vi "Normal.vi"() -> (0 "高難度挑戰":bool)   [LabVIEW 2014]
uses:
  <vilib>/Utility/inputDevices.llb/keyboardAcquire.vi
  <vilib>/Utility/inputDevices.llb/closeKeyboard.vi
panel:
  out "Å]YÄ²":i32
  out "Å]XÄ²":i32
  out "Å]Vy":i64
  out "Å]Vx":i32
  out "魔王":bool
  out "終點":bool
  out "遊玩時間":i32
  out "X障礙":bool
  out "Y位置 2":i32
  out "x位置 2":i32
  out "X":dbl
  out "Y":dbl
  out "小精靈":bool
  out "x位置":i32
  out "Y位置":i32
  out "Y障礙":bool
  out "x觸及位置":i32
  out "y觸及位置":i32
  out "x-y":u32
  out "Vy":i32
  out "Vx":i32
  # "小精靈"
  # "500"
  # "障礙"
  # "400"
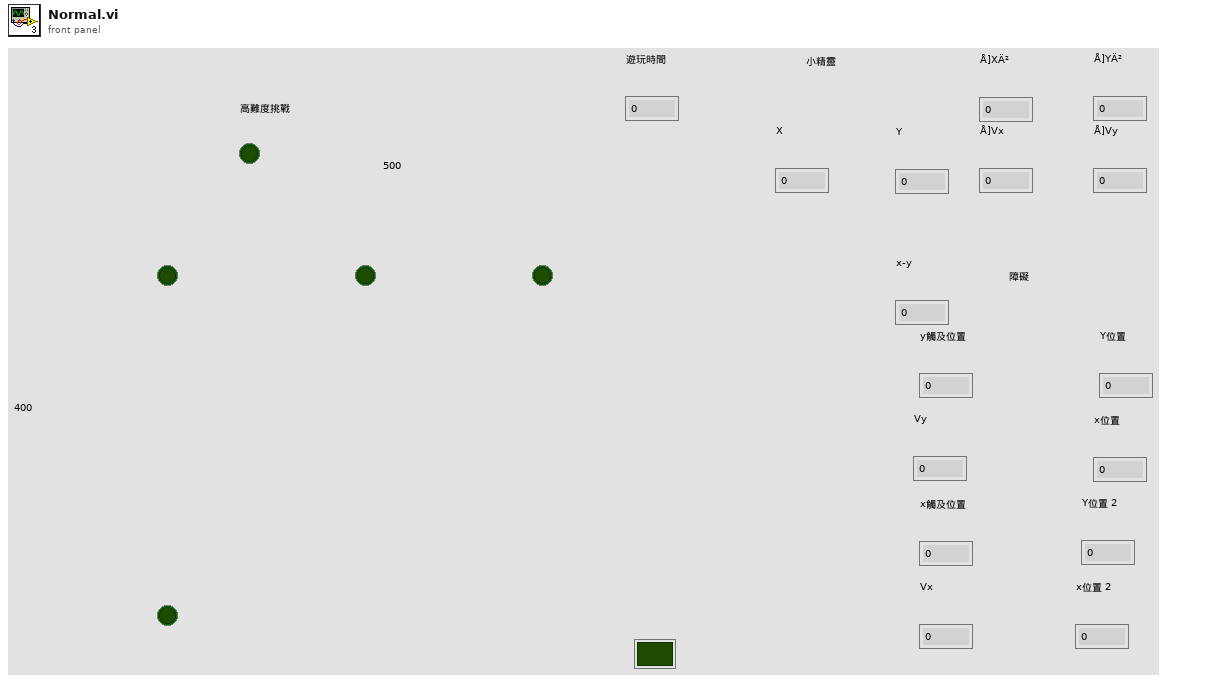
[diagram p1: front panel]
types:
  T1 = enum16{"0", "1", "2", "3", "4", "5", "6", "7", "8", "9", "A", "B", "C", "D", "E", "F", "G", "H", "I", "J", "K", "L", "M", "N", "O", "P", "Q", "R", "S", "T", "U", "V", "W", "X", "Y", "Z", "F1", "F2", "F3", "F4", "F5", "F6", "F7", "F8", "F9", "F10", "F11", "F12", "F13", "F14", "F15", "ADD", "BACK", "BACKSLASH", "CAPITAL", "COMMA", "DECIMAL", "DELETE", "DIVIDE", "DOWN", "END", "EQUALS", "ESCAPE", "GRAVE (`)", "HOME", "INSERT", "LBRACKET", "LCONTROL", "LEFT", "L ALT", "LSHIFT", "LWIN", "MINUS", "MULTIPLY", "NEXT", "NUMLOCK", "NUMPAD_0", "NUMPAD_1", "NUMPAD_2", "NUMPAD_3", "NUMPAD_4", "NUMPAD_5", "NUMPAD_6", "NUMPAD_7", "NUMPAD_8", "NUMPAD_9", "PAUSE", "PERIOD", "PRIOR (PG UP)", "RBRACKET", "RCONTROL", "RETURN", "RIGHT", "R ALT", "RSHIFT", "RWIN", "SCROLL", "SEMICOLON", "SLASH", "SPACE", "SUBTRACT", "TAB", "UP", "ENTER (num pad)", "' (quote)"}[]
  T2 = cluster{"keys pressed[0]":enum16{"0", "1", "2", "3", "4", "5", "6", "7", "8", "9", "A", "B", "C", "D", "E", "F", "G", "H", "I", "J", "K", "L", "M", "N", "O", "P", "Q", "R", "S", "T", "U", "V", "W", "X", "Y", "Z", "F1", "F2", "F3", "F4", "F5", "F6", "F7", "F8", "F9", "F10", "F11", "F12", "F13", "F14", "F15", "ADD", "BACK", "BACKSLASH", "CAPITAL", "COMMA", "DECIMAL", "DELETE", "DIVIDE", "DOWN", "END", "EQUALS", "ESCAPE", "GRAVE (`)", "HOME", "INSERT", "LBRACKET", "LCONTROL", "LEFT", "L ALT", "LSHIFT", "LWIN", "MINUS", "MULTIPLY", "NEXT", "NUMLOCK", "NUMPAD_0", "NUMPAD_1", "NUMPAD_2", "NUMPAD_3", "NUMPAD_4", "NUMPAD_5", "NUMPAD_6", "NUMPAD_7", "NUMPAD_8", "NUMPAD_9", "PAUSE", "PERIOD", "PRIOR (PG UP)", "RBRACKET", "RCONTROL", "RETURN", "RIGHT", "R ALT", "RSHIFT", "RWIN", "SCROLL", "SEMICOLON", "SLASH", "SPACE", "SUBTRACT", "TAB", "UP", "ENTER (num pad)", "' (quote)"}, "keys pressed[1]":enum16{"0", "1", "2", "3", "4", "5", "6", "7", "8", "9", "A", "B", "C", "D", "E", "F", "G", "H", "I", "J", "K", "L", "M", "N", "O", "P", "Q", "R", "S", "T", "U", "V", "W", "X", "Y", "Z", "F1", "F2", "F3", "F4", "F5", "F6", "F7", "F8", "F9", "F10", "F11", "F12", "F13", "F14", "F15", "ADD", "BACK", "BACKSLASH", "CAPITAL", "COMMA", "DECIMAL", "DELETE", "DIVIDE", "DOWN", "END", "EQUALS", "ESCAPE", "GRAVE (`)", "HOME", "INSERT", "LBRACKET", "LCONTROL", "LEFT", "L ALT", "LSHIFT", "LWIN", "MINUS", "MULTIPLY", "NEXT", "NUMLOCK", "NUMPAD_0", "NUMPAD_1", "NUMPAD_2", "NUMPAD_3", "NUMPAD_4", "NUMPAD_5", "NUMPAD_6", "NUMPAD_7", "NUMPAD_8", "NUMPAD_9", "PAUSE", "PERIOD", "PRIOR (PG UP)", "RBRACKET", "RCONTROL", "RETURN", "RIGHT", "R ALT", "RSHIFT", "RWIN", "SCROLL", "SEMICOLON", "SLASH", "SPACE", "SUBTRACT", "TAB", "UP", "ENTER (num pad)", "' (quote)"}, "keys pressed[2]":enum16{"0", "1", "2", "3", "4", "5", "6", "7", "8", "9", "A", "B", "C", "D", "E", "F", "G", "H", "I", "J", "K", "L", "M", "N", "O", "P", "Q", "R", "S", "T", "U", "V", "W", "X", "Y", "Z", "F1", "F2", "F3", "F4", "F5", "F6", "F7", "F8", "F9", "F10", "F11", "F12", "F13", "F14", "F15", "ADD", "BACK", "BACKSLASH", "CAPITAL", "COMMA", "DECIMAL", "DELETE", "DIVIDE", "DOWN", "END", "EQUALS", "ESCAPE", "GRAVE (`)", "HOME", "INSERT", "LBRACKET", "LCONTROL", "LEFT", "L ALT", "LSHIFT", "LWIN", "MINUS", "MULTIPLY", "NEXT", "NUMLOCK", "NUMPAD_0", "NUMPAD_1", "NUMPAD_2", "NUMPAD_3", "NUMPAD_4", "NUMPAD_5", "NUMPAD_6", "NUMPAD_7", "NUMPAD_8", "NUMPAD_9", "PAUSE", "PERIOD", "PRIOR (PG UP)", "RBRACKET", "RCONTROL", "RETURN", "RIGHT", "R ALT", "RSHIFT", "RWIN", "SCROLL", "SEMICOLON", "SLASH", "SPACE", "SUBTRACT", "TAB", "UP", "ENTER (num pad)", "' (quote)"}, "keys pressed[3]":enum16{"0", "1", "2", "3", "4", "5", "6", "7", "8", "9", "A", "B", "C", "D", "E", "F", "G", "H", "I", "J", "K", "L", "M", "N", "O", "P", "Q", "R", "S", "T", "U", "V", "W", "X", "Y", "Z", "F1", "F2", "F3", "F4", "F5", "F6", "F7", "F8", "F9", "F10", "F11", "F12", "F13", "F14", "F15", "ADD", "BACK", "BACKSLASH", "CAPITAL", "COMMA", "DECIMAL", "DELETE", "DIVIDE", "DOWN", "END", "EQUALS", "ESCAPE", "GRAVE (`)", "HOME", "INSERT", "LBRACKET", "LCONTROL", "LEFT", "L ALT", "LSHIFT", "LWIN", "MINUS", "MULTIPLY", "NEXT", "NUMLOCK", "NUMPAD_0", "NUMPAD_1", "NUMPAD_2", "NUMPAD_3", "NUMPAD_4", "NUMPAD_5", "NUMPAD_6", "NUMPAD_7", "NUMPAD_8", "NUMPAD_9", "PAUSE", "PERIOD", "PRIOR (PG UP)", "RBRACKET", "RCONTROL", "RETURN", "RIGHT", "R ALT", "RSHIFT", "RWIN", "SCROLL", "SEMICOLON", "SLASH", "SPACE", "SUBTRACT", "TAB", "UP", "ENTER (num pad)", "' (quote)"}, "keys pressed[4]":enum16{"0", "1", "2", "3", "4", "5", "6", "7", "8", "9", "A", "B", "C", "D", "E", "F", "G", "H", "I", "J", "K", "L", "M", "N", "O", "P", "Q", "R", "S", "T", "U", "V", "W", "X", "Y", "Z", "F1", "F2", "F3", "F4", "F5", "F6", "F7", "F8", "F9", "F10", "F11", "F12", "F13", "F14", "F15", "ADD", "BACK", "BACKSLASH", "CAPITAL", "COMMA", "DECIMAL", "DELETE", "DIVIDE", "DOWN", "END", "EQUALS", "ESCAPE", "GRAVE (`)", "HOME", "INSERT", "LBRACKET", "LCONTROL", "LEFT", "L ALT", "LSHIFT", "LWIN", "MINUS", "MULTIPLY", "NEXT", "NUMLOCK", "NUMPAD_0", "NUMPAD_1", "NUMPAD_2", "NUMPAD_3", "NUMPAD_4", "NUMPAD_5", "NUMPAD_6", "NUMPAD_7", "NUMPAD_8", "NUMPAD_9", "PAUSE", "PERIOD", "PRIOR (PG UP)", "RBRACKET", "RCONTROL", "RETURN", "RIGHT", "R ALT", "RSHIFT", "RWIN", "SCROLL", "SEMICOLON", "SLASH", "SPACE", "SUBTRACT", "TAB", "UP", "ENTER (num pad)", "' (quote)"}, "keys pressed[5]":enum16{"0", "1", "2", "3", "4", "5", "6", "7", "8", "9", "A", "B", "C", "D", "E", "F", "G", "H", "I", "J", "K", "L", "M", "N", "O", "P", "Q", "R", "S", "T", "U", "V", "W", "X", "Y", "Z", "F1", "F2", "F3", "F4", "F5", "F6", "F7", "F8", "F9", "F10", "F11", "F12", "F13", "F14", "F15", "ADD", "BACK", "BACKSLASH", "CAPITAL", "COMMA", "DECIMAL", "DELETE", "DIVIDE", "DOWN", "END", "EQUALS", "ESCAPE", "GRAVE (`)", "HOME", "INSERT", "LBRACKET", "LCONTROL", "LEFT", "L ALT", "LSHIFT", "LWIN", "MINUS", "MULTIPLY", "NEXT", "NUMLOCK", "NUMPAD_0", "NUMPAD_1", "NUMPAD_2", "NUMPAD_3", "NUMPAD_4", "NUMPAD_5", "NUMPAD_6", "NUMPAD_7", "NUMPAD_8", "NUMPAD_9", "PAUSE", "PERIOD", "PRIOR (PG UP)", "RBRACKET", "RCONTROL", "RETURN", "RIGHT", "R ALT", "RSHIFT", "RWIN", "SCROLL", "SEMICOLON", "SLASH", "SPACE", "SUBTRACT", "TAB", "UP", "ENTER (num pad)", "' (quote)"}, "keys pressed[6]":enum16{"0", "1", "2", "3", "4", "5", "6", "7", "8", "9", "A", "B", "C", "D", "E", "F", "G", "H", "I", "J", "K", "L", "M", "N", "O", "P", "Q", "R", "S", "T", "U", "V", "W", "X", "Y", "Z", "F1", "F2", "F3", "F4", "F5", "F6", "F7", "F8", "F9", "F10", "F11", "F12", "F13", "F14", "F15", "ADD", "BACK", "BACKSLASH", "CAPITAL", "COMMA", "DECIMAL", "DELETE", "DIVIDE", "DOWN", "END", "EQUALS", "ESCAPE", "GRAVE (`)", "HOME", "INSERT", "LBRACKET", "LCONTROL", "LEFT", "L ALT", "LSHIFT", "LWIN", "MINUS", "MULTIPLY", "NEXT", "NUMLOCK", "NUMPAD_0", "NUMPAD_1", "NUMPAD_2", "NUMPAD_3", "NUMPAD_4", "NUMPAD_5", "NUMPAD_6", "NUMPAD_7", "NUMPAD_8", "NUMPAD_9", "PAUSE", "PERIOD", "PRIOR (PG UP)", "RBRACKET", "RCONTROL", "RETURN", "RIGHT", "R ALT", "RSHIFT", "RWIN", "SCROLL", "SEMICOLON", "SLASH", "SPACE", "SUBTRACT", "TAB", "UP", "ENTER (num pad)", "' (quote)"}, "keys pressed[7]":enum16{"0", "1", "2", "3", "4", "5", "6", "7", "8", "9", "A", "B", "C", "D", "E", "F", "G", "H", "I", "J", "K", "L", "M", "N", "O", "P", "Q", "R", "S", "T", "U", "V", "W", "X", "Y", "Z", "F1", "F2", "F3", "F4", "F5", "F6", "F7", "F8", "F9", "F10", "F11", "F12", "F13", "F14", "F15", "ADD", "BACK", "BACKSLASH", "CAPITAL", "COMMA", "DECIMAL", "DELETE", "DIVIDE", "DOWN", "END", "EQUALS", "ESCAPE", "GRAVE (`)", "HOME", "INSERT", "LBRACKET", "LCONTROL", "LEFT", "L ALT", "LSHIFT", "LWIN", "MINUS", "MULTIPLY", "NEXT", "NUMLOCK", "NUMPAD_0", "NUMPAD_1", "NUMPAD_2", "NUMPAD_3", "NUMPAD_4", "NUMPAD_5", "NUMPAD_6", "NUMPAD_7", "NUMPAD_8", "NUMPAD_9", "PAUSE", "PERIOD", "PRIOR (PG UP)", "RBRACKET", "RCONTROL", "RETURN", "RIGHT", "R ALT", "RSHIFT", "RWIN", "SCROLL", "SEMICOLON", "SLASH", "SPACE", "SUBTRACT", "TAB", "UP", "ENTER (num pad)", "' (quote)"}, "keys pressed[8]":enum16{"0", "1", "2", "3", "4", "5", "6", "7", "8", "9", "A", "B", "C", "D", "E", "F", "G", "H", "I", "J", "K", "L", "M", "N", "O", "P", "Q", "R", "S", "T", "U", "V", "W", "X", "Y", "Z", "F1", "F2", "F3", "F4", "F5", "F6", "F7", "F8", "F9", "F10", "F11", "F12", "F13", "F14", "F15", "ADD", "BACK", "BACKSLASH", "CAPITAL", "COMMA", "DECIMAL", "DELETE", "DIVIDE", "DOWN", "END", "EQUALS", "ESCAPE", "GRAVE (`)", "HOME", "INSERT", "LBRACKET", "LCONTROL", "LEFT", "L ALT", "LSHIFT", "LWIN", "MINUS", "MULTIPLY", "NEXT", "NUMLOCK", "NUMPAD_0", "NUMPAD_1", "NUMPAD_2", "NUMPAD_3", "NUMPAD_4", "NUMPAD_5", "NUMPAD_6", "NUMPAD_7", "NUMPAD_8", "NUMPAD_9", "PAUSE", "PERIOD", "PRIOR (PG UP)", "RBRACKET", "RCONTROL", "RETURN", "RIGHT", "R ALT", "RSHIFT", "RWIN", "SCROLL", "SEMICOLON", "SLASH", "SPACE", "SUBTRACT", "TAB", "UP", "ENTER (num pad)", "' (quote)"}}
  T3 = enum16{"0", "1", "2", "3", "4", "5", "6", "7", "8", "9", "A", "B", "C", "D", "E", "F", "G", "H", "I", "J", "K", "L", "M", "N", "O", "P", "Q", "R", "S", "T", "U", "V", "W", "X", "Y", "Z", "F1", "F2", "F3", "F4", "F5", "F6", "F7", "F8", "F9", "F10", "F11", "F12", "F13", "F14", "F15", "ADD", "BACK", "BACKSLASH", "CAPITAL", "COMMA", "DECIMAL", "DELETE", "DIVIDE", "DOWN", "END", "EQUALS", "ESCAPE", "GRAVE (`)", "HOME", "INSERT", "LBRACKET", "LCONTROL", "LEFT", "L ALT", "LSHIFT", "LWIN", "MINUS", "MULTIPLY", "NEXT", "NUMLOCK", "NUMPAD_0", "NUMPAD_1", "NUMPAD_2", "NUMPAD_3", "NUMPAD_4", "NUMPAD_5", "NUMPAD_6", "NUMPAD_7", "NUMPAD_8", "NUMPAD_9", "PAUSE", "PERIOD", "PRIOR (PG UP)", "RBRACKET", "RCONTROL", "RETURN", "RIGHT", "R ALT", "RSHIFT", "RWIN", "SCROLL", "SEMICOLON", "SLASH", "SPACE", "SUBTRACT", "TAB", "UP", "ENTER (num pad)", "' (quote)"}
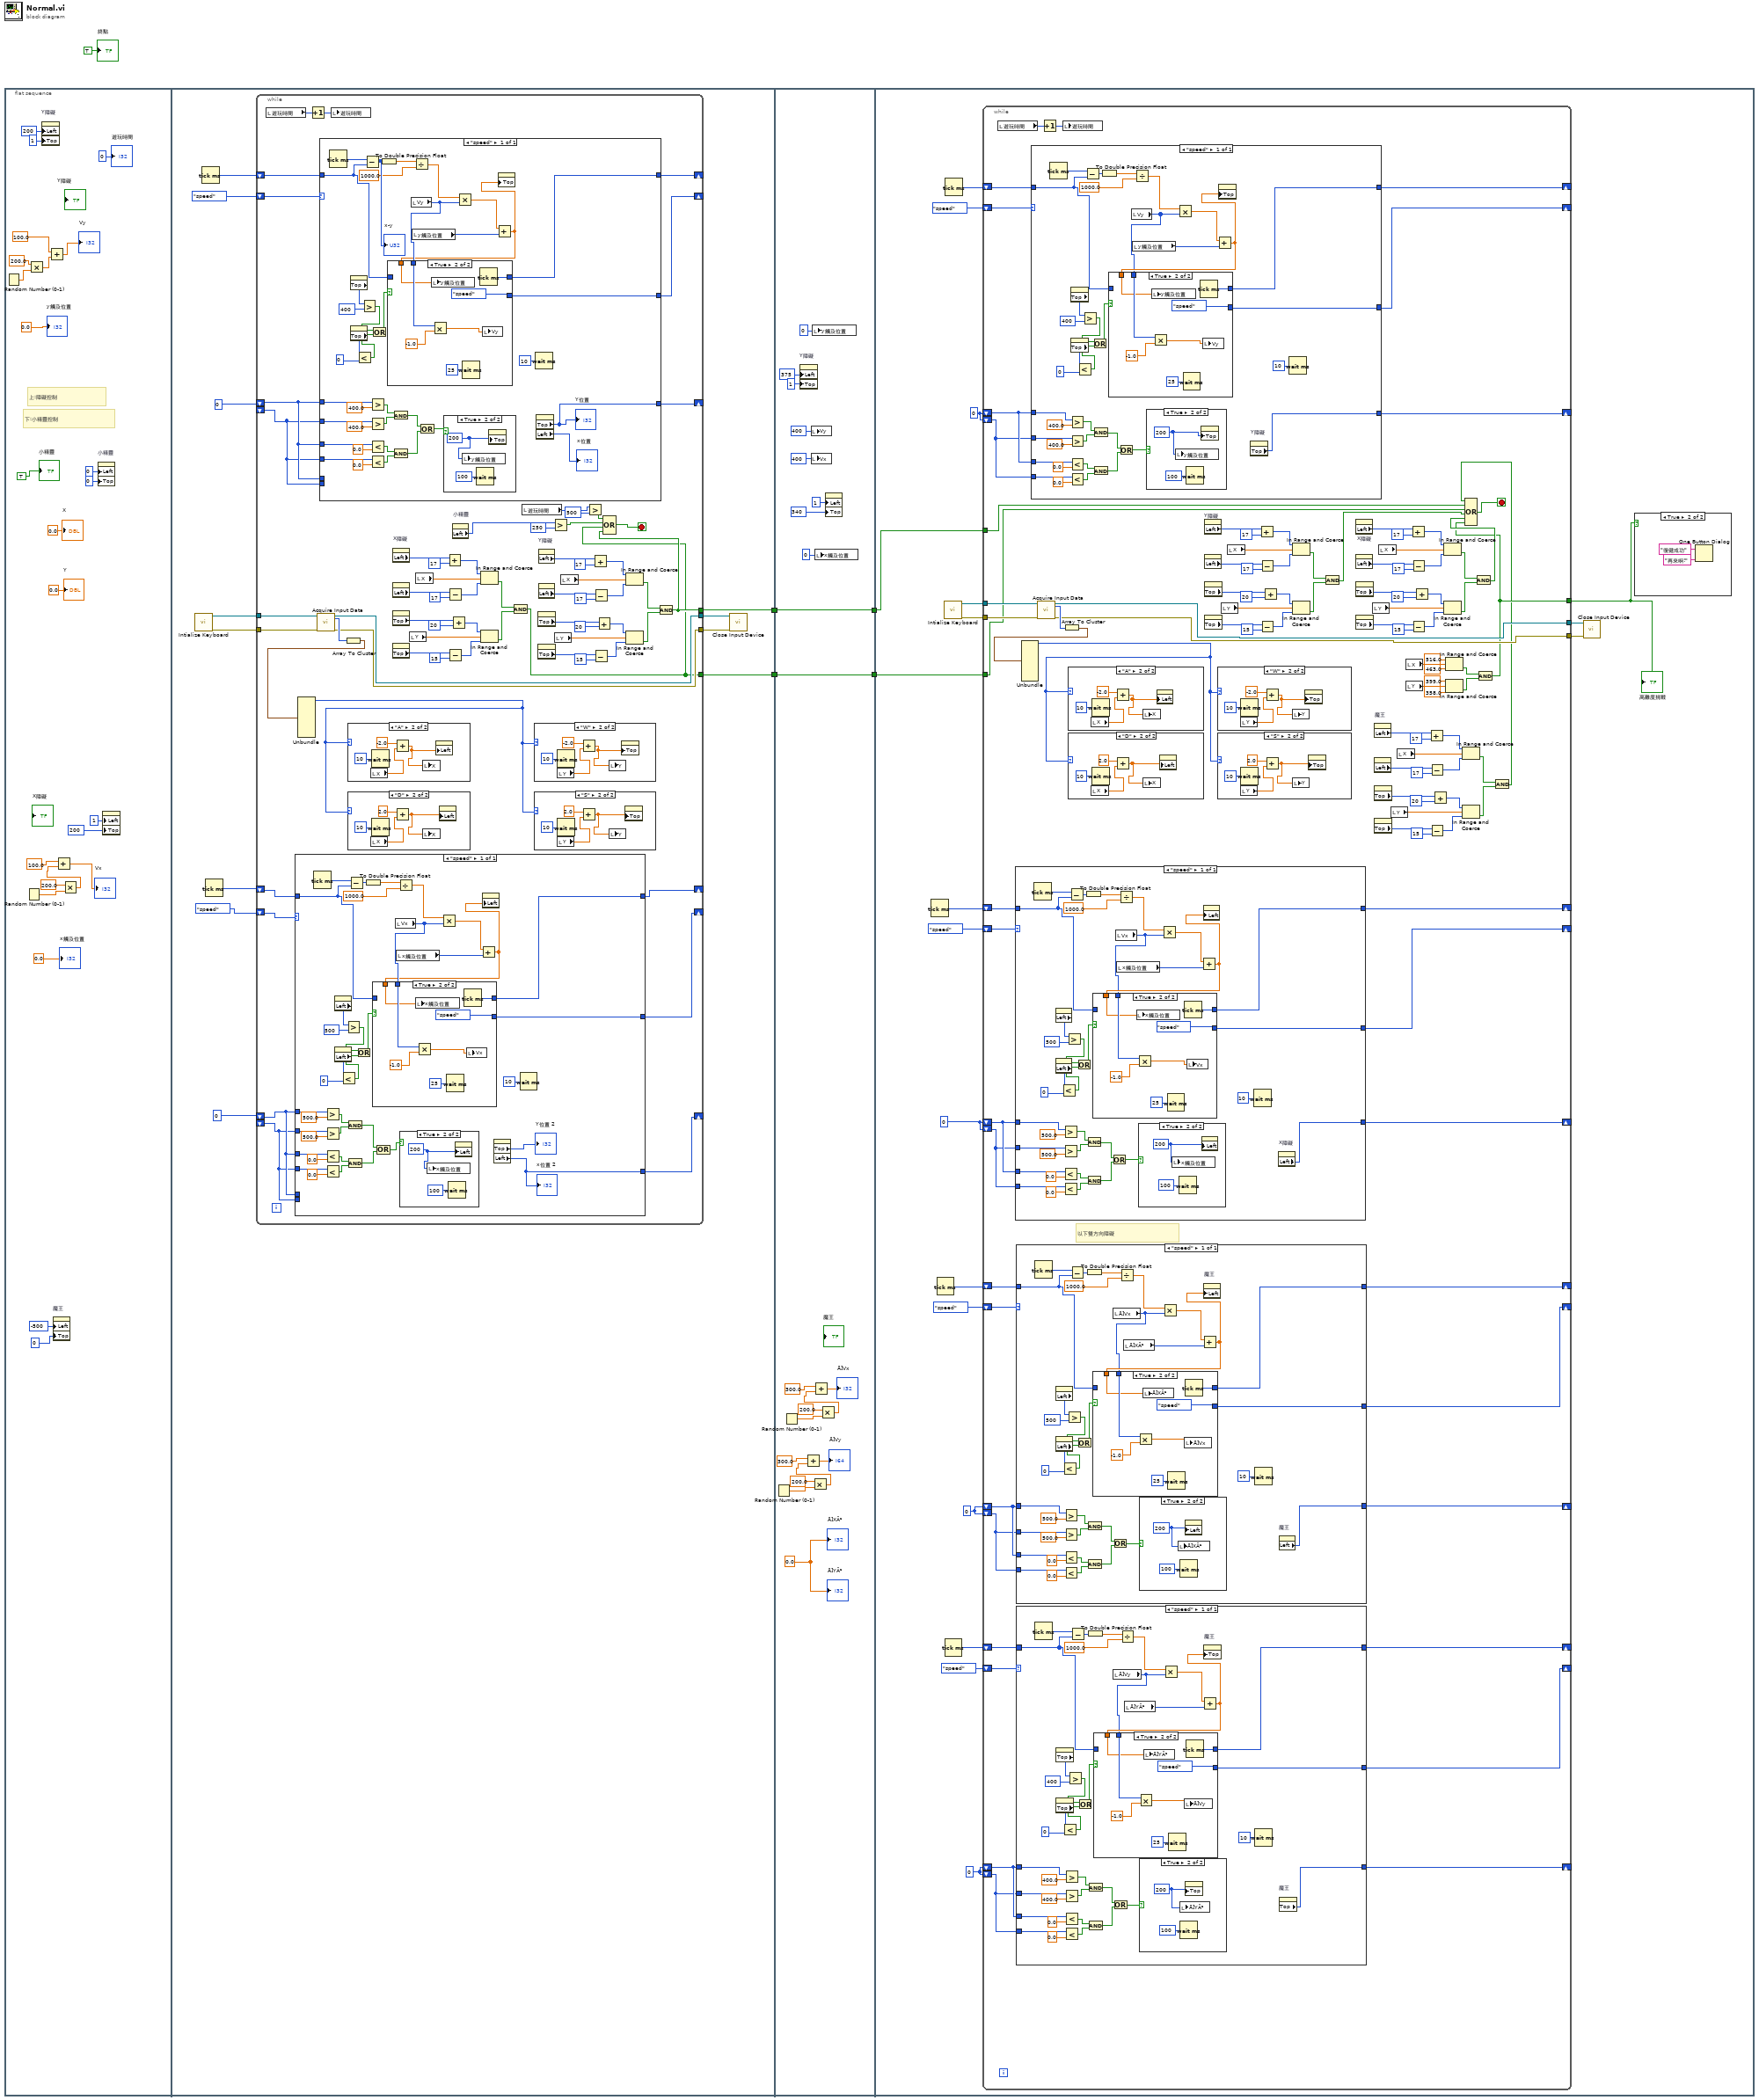
[diagram p0: block diagram]
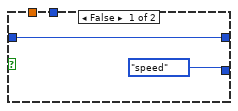
[diagram p3: hidden frame]
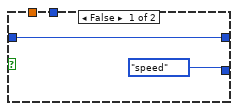
[diagram p9: hidden frame]
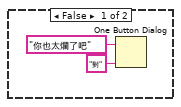
[diagram p10: hidden frame]
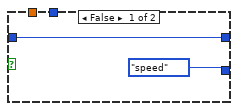
[diagram p12: hidden frame]
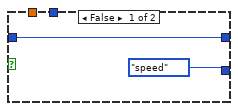
[diagram p14: hidden frame]
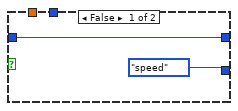
[diagram p16: hidden frame]
diagram:
  n1 = flat-sequence {
    tunnel: [w31] -> w4
    tunnel: [w30] -> w2
    tunnel: [w230] -> w5
    tunnel: w4 -> [w230]
    tunnel: [w229] -> w3
    tunnel: w2 -> [w229]
    tunnel: w5 -> [w249]
    tunnel: w3 -> [w248]
    frame #0 {
      # "下:小精靈控制"
      # "上:障礙控制"
      n2 = Random Number (0-1)() -> (number: 0 to 1=w19:dbl)
      n3 = Random Number (0-1)() -> (number: 0 to 1=w24:dbl)
      n4 = Multiply(x=200.0, y=w19) -> (x*y=w17:dbl)
      n5 = property on="Y障礙" class="Bool (strict)"("Left"=200 ("Position:Left"), "Top"=1 ("Position:Top")) -> ()  [unwired: 2 in, 2 out]
      n6 = Add(x=100.0 ("Vy"), y=w17) -> (x+y=→"Vy":dbl)
      n7 = property on="魔王" class="Bool (strict)"("Left"=-500 ("Position:Left"), "Top"=0 ("Position:Top")) -> ()  [unwired: 2 in, 2 out]
      n8 = Multiply(x=200.0, y=w24) -> (x*y=w22:dbl)
      n9 = Add(x=100.0 ("y"), y=w22) -> (x+y=→"Vx":dbl)
      n10 = property on="小精靈" class="Bool (strict)"("Left"=0 ("Position:Left"), "Top"=0 ("Position:Top")) -> ()  [unwired: 2 in, 2 out]
      n11 = property on="X障礙" class="Bool (strict)"("Left"=1 ("Position:Left"), "Top"=200 ("Position:Top")) -> ()  [unwired: 2 in, 2 out]
      "y觸及位置" <- 0.0 ("x*y")
      "x觸及位置" <- 0.0 ("x*y")
      "小精靈" <- TRUE
      "X" <- 0.0 ("Numeric")
      "Y" <- 0.0 ("Y")
      "遊玩時間" <- 0 ("Numeric")
    }
    frame #1 {
      w32 = 0
      w33 = 0
      n12 = call <vilib>:"Intialize Keyboard.vi"() -> ("error out"=w37:errorcluster, "device ID"=w39:refnum<k1>)  [unwired: 10 in]
      n13 = Tick Count (ms)() -> (millisecond timer value=w40:u32)
      n14 = Tick Count (ms)() -> (millisecond timer value=w35:u32)
      n15 = while {
        shift-right: [w102] -> _
        shift-left: enum16{"speed"}."speed" ("Enum") -> [w104]
        shift-right: [w103] -> _
        shift-left: w40 -> [w105]
        tunnel: w39 -> [w101]
        tunnel: [w68] -> w38
        tunnel: w37 -> [w100]
        tunnel: [w67] -> w36
        shift-right: [w96] -> _
        shift-left: w35 -> [w97]
        shift-right: [w95] -> _
        shift-left: enum16{"speed"}."speed" ("Enum") -> [w94]
        shift-right: [w91] -> _
        shift-left: w33 -> [w89]
        shift-left: w33 -> [w88]
        shift-right: [w90] -> _
        shift-left: w32 -> [w87]
        shift-left: w32 -> [w86]
        tunnel: [w49] -> w31
        tunnel: [w48] -> w30
        stop <- w47 stop-if-true
        n16 = local read "遊玩時間"() -> (w46:i32)
        n17 = case shown="\"speed\"" w94 {
          tunnel: w97 -> [w133]
          tunnel: [w132] -> w96
          tunnel: [w131] -> w95
          tunnel: w89 -> [w121]
          tunnel: w88 -> [w120]
          tunnel: w89 -> [w115]
          tunnel: w88 -> [w114]
          tunnel: [w109] -> w91
          tunnel: w89 -> [_]
          tunnel: w88 -> [_]
          frame "speed" {
            n18 = Tick Count (ms)() -> (millisecond timer value=w142:u32)
            n19 = Greater?(x=w121, y=500.0) -> (0:w117:bool)
            n20 = Greater?(x=w120, y=500.0) -> (0:w116:bool)
            n21 = Less?(x=w115, y=0.0) -> (x < y?=w111:bool)
            n22 = Less?(x=w114, y=0.0) -> (x < y?=w110:bool)
            n23 = property on="X障礙" class="Bool (strict)"() -> ("Left"=w134:i32)  [unwired: 2 in, 2 out]
            n24 = property on="X障礙" class="Bool (strict)"() -> ("Left"=w128:i32)  [unwired: 2 in, 2 out]
            n25 = Less?(x=w128, y=0) -> (x < y?=w126:bool)
            n26 = Greater?(x=w134, y=500) -> (0:w125:bool)
            n27 = And(x=w117, y=w116) -> (x .and. y?=w108:bool)
            n28 = And(x=w111, y=w110) -> (x .and. y?=w107:bool)
            n29 = Subtract(x=w142, y=w133) -> (x-y=w141:u32)
            n30 = Or(x=w125, y=w126) -> (x .or. y?=w124:bool)
            n31 = To Double Precision Float(number=w141) -> (double precision float=w140:dbl)
            n32 = Compound Arithmetic op=OR(w108, w107) -> (w106:bool)
            n33 = local read "Vx"() -> (w130:i32)
            n34 = local read "x觸及位置"() -> (w136:i32)
            n35 = Divide(x=w140, y=1000.0) -> (x/y=w138:dbl)
            n36 = case shown="True" w106 {
              frame False {
              }
              frame True {
                w143 = 200 ("x觸及位置")
                n37 = local write "x觸及位置"(w143) -> ()
                n38 = Wait (ms)(milliseconds to wait=u32 100) -> ()  [unwired: 1 out]
                n39 = property on="X障礙" class="Bool (strict)"("Left"=w143) -> ()  [unwired: 2 in, 2 out]
              }
            }
            n40 = Multiply(x=w138, y=w130) -> (x*y=w137:dbl)
            n41 = Add(x=w137, y=w136) -> (x+y=w122:dbl)
            n42 = case shown="True" w124 {
              tunnel: [enum16{"speed"}."speed" ("Enum") enum16{"speed"}."speed" ("Enum")] -> w131
              tunnel: [w145 w152] -> w132
              tunnel: w133 -> [w145 _]
              tunnel: w122 -> [_ w149]
              tunnel: w130 -> [_ w151]
              frame False {
              }
              frame True {
                n43 = local write "x觸及位置"(w149) -> ()
                n44 = Multiply(x=w151, y=-1.0) -> (x*y=w148:dbl)
                n45 = Wait (ms)(milliseconds to wait=u32 25) -> ()  [unwired: 1 out]
                n46 = Tick Count (ms)() -> (millisecond timer value=w152:u32)
                n47 = local write "Vx"(w148) -> ()
              }
            }
            n48 = property on="X障礙" class="Bool (strict)"("Left"=w122) -> ()  [unwired: 2 in, 2 out]
            n49 = property on="X障礙" class="Bool (strict)"() -> ("Top"=→"Y位置 2":i32, "Left"=w109:i32)  [unwired: 2 in, 2 out]
            "x位置 2" <- w109
            n50 = Wait (ms)(milliseconds to wait=u32 10) -> ()  [unwired: 1 out]
          }
        }
        n51 = Increment(x=w46) -> (x+1=w45:i32)
        n52 = call-poly <vilib>:"Acquire Input Data.vi"("device ID"=w101, "error in (no error)"=w100) -> ("device ID"=w68:refnum<k1>, "keys pressed"=w99:T1, "error out"=w67:errorcluster)  [unwired: 15 in]
        n53 = case shown="\"speed\"" w104 {
          tunnel: w105 -> [w197]
          tunnel: [w196] -> w103
          tunnel: [w195] -> w102
          tunnel: w87 -> [w177]
          tunnel: w87 -> [w176]
          tunnel: w86 -> [w175]
          tunnel: w86 -> [w174]
          tunnel: [w173] -> w90
          tunnel: w87 -> [_]
          tunnel: w86 -> [_]
          frame "speed" {
            n54 = Tick Count (ms)() -> (millisecond timer value=w206:u32)
            n55 = property on="Y障礙" class="Bool (strict)"() -> ("Top"=w198:i32)  [unwired: 2 in, 2 out]
            n56 = property on="Y障礙" class="Bool (strict)"() -> ("Top"=w192:i32)  [unwired: 2 in, 2 out]
            n57 = Less?(x=w192, y=0) -> (x < y?=w190:bool)
            n58 = Greater?(x=w198, y=400) -> (0:w189:bool)
            n59 = Subtract(x=w206, y=w197) -> (x-y=w205:u32)
            "x-y" <- w205
            n60 = Greater?(x=w177, y=400.0) -> (0:w183:bool)
            n61 = Greater?(x=w175, y=400.0) -> (0:w182:bool)
            n62 = Less?(x=w176, y=0.0) -> (x < y?=w179:bool)
            n63 = Less?(x=w174, y=0.0) -> (x < y?=w178:bool)
            n64 = Or(x=w189, y=w190) -> (x .or. y?=w188:bool)
            n65 = To Double Precision Float(number=w205) -> (double precision float=w204:dbl)
            n66 = And(x=w183, y=w182) -> (x .and. y?=w172:bool)
            n67 = And(x=w179, y=w178) -> (x .and. y?=w171:bool)
            n68 = local read "Vy"() -> (w194:i32)
            n69 = local read "y觸及位置"() -> (w200:i32)
            n70 = Divide(x=w204, y=1000.0) -> (x/y=w202:dbl)
            n71 = Compound Arithmetic op=OR(w172, w171) -> (w170:bool)
            n72 = case shown="True" w170 {
              frame False {
              }
              frame True {
                w207 = 200 ("y觸及位置")
                n73 = local write "y觸及位置"(w207) -> ()
                n74 = Wait (ms)(milliseconds to wait=u32 100) -> ()  [unwired: 1 out]
                n75 = property on="Y障礙" class="Bool (strict)"("Top"=w207) -> ()  [unwired: 2 in, 2 out]
              }
            }
            n76 = Multiply(x=w202, y=w194) -> (x*y=w201:dbl)
            n77 = Add(x=w201, y=w200) -> (x+y=w186:dbl)
            n78 = case shown="True" w188 {
              tunnel: [enum16{"speed"}."speed" ("Enum") enum16{"speed"}."speed" ("Enum")] -> w195
              tunnel: [w209 w216] -> w196
              tunnel: w197 -> [w209 _]
              tunnel: w186 -> [_ w212]
              tunnel: w194 -> [_ w214]
              frame False {
              }
              frame True {
                n79 = local write "y觸及位置"(w212) -> ()
                n80 = Multiply(x=w214, y=-1.0) -> (x*y=w211:dbl)
                n81 = Wait (ms)(milliseconds to wait=u32 25) -> ()  [unwired: 1 out]
                n82 = Tick Count (ms)() -> (millisecond timer value=w216:u32)
                n83 = local write "Vy"(w211) -> ()
              }
            }
            n84 = property on="Y障礙" class="Bool (strict)"("Top"=w186) -> ()  [unwired: 2 in, 2 out]
            n85 = Wait (ms)(milliseconds to wait=u32 10) -> ()  [unwired: 1 out]
            n86 = property on="Y障礙" class="Bool (strict)"() -> ("Top"=w173:i32, "Left"=→"x位置":i32)  [unwired: 2 in, 2 out]
            "Y位置" <- w173
          }
        }
        n87 = local write "遊玩時間"(w45) -> ()
        n88 = Array To Cluster(array=w99) -> (cluster=w69:T2)
        n89 = Unbundle(w69) -> ("keys pressed[0]"=w98:T3)  [unwired: 8 out]
        n90 = case shown="\"A\"" w98 {
          frame Default {
          }
          frame "A" {
            n91 = local read "X"() -> (w168:dbl)
            n92 = Wait (ms)(milliseconds to wait=u32 10) -> ()  [unwired: 1 out]
            n93 = Add(x=-2.0, y=w168) -> (x+y=w166:dbl)
            n94 = local write "X"(w166) -> ()
            n95 = property on="小精靈" class="Bool (strict)"("Left"=w166) -> ()  [unwired: 2 in, 2 out]
          }
        }
        n96 = case shown="\"D\"" w98 {
          frame Default {
          }
          frame "D" {
            n97 = local read "X"() -> (w164:dbl)
            n98 = Wait (ms)(milliseconds to wait=u32 10) -> ()  [unwired: 1 out]
            n99 = Add(x=2.0, y=w164) -> (x+y=w162:dbl)
            n100 = local write "X"(w162) -> ()
            n101 = property on="小精靈" class="Bool (strict)"("Left"=w162) -> ()  [unwired: 2 in, 2 out]
          }
        }
        n102 = property on="X障礙" class="Bool (strict)"() -> ("Top"=w66:i32)  [unwired: 2 in, 2 out]
        n103 = property on="X障礙" class="Bool (strict)"() -> ("Top"=w60:i32)  [unwired: 2 in, 2 out]
        n104 = property on="X障礙" class="Bool (strict)"() -> ("Left"=w53:i32)  [unwired: 2 in, 2 out]
        n105 = property on="X障礙" class="Bool (strict)"() -> ("Left"=w55:i32)  [unwired: 2 in, 2 out]
        n106 = local read "Y"() -> (w52:dbl)
        n107 = local read "X"() -> (w51:dbl)
        n108 = Add(x=w53, y=17) -> (x+y=w58:i32)
        n109 = Subtract(x=w55, y=17) -> (x-y=w57:i32)
        n110 = Subtract(x=w60, y=15) -> (x-y=w61:i32)
        n111 = Add(x=w66, y=20) -> (x+y=w65:i32)
        n112 = property on="小精靈" class="Bool (strict)"() -> ("Left"=w93:i32)  [unwired: 2 in, 2 out]
        n113 = In Range and Coerce(upper limit=w58, x=w51, lower limit=w57) -> (In Range?=w62:bool)  [unwired: 1 out]
        n114 = In Range and Coerce(upper limit=w65, x=w52, lower limit=w61) -> (In Range?=w63:bool)  [unwired: 1 out]
        n115 = And(x=w62, y=w63) -> (x .and. y?=w48:bool)
        n116 = local read "遊玩時間"() -> (w44:i32)
        n117 = case shown="\"W\"" w98 {
          frame Default {
          }
          frame "W" {
            n118 = local read "Y"() -> (w160:dbl)
            n119 = Wait (ms)(milliseconds to wait=u32 10) -> ()  [unwired: 1 out]
            n120 = Add(x=-2.0, y=w160) -> (x+y=w158:dbl)
            n121 = local write "Y"(w158) -> ()
            n122 = property on="小精靈" class="Bool (strict)"("Top"=w158) -> ()  [unwired: 2 in, 2 out]
          }
        }
        n123 = case shown="\"S\"" w98 {
          frame Default {
          }
          frame "S" {
            n124 = local read "Y"() -> (w156:dbl)
            n125 = Wait (ms)(milliseconds to wait=u32 10) -> ()  [unwired: 1 out]
            n126 = Add(x=2.0, y=w156) -> (x+y=w154:dbl)
            n127 = local write "Y"(w154) -> ()
            n128 = property on="小精靈" class="Bool (strict)"("Top"=w154) -> ()  [unwired: 2 in, 2 out]
          }
        }
        n129 = property on="Y障礙" class="Bool (strict)"() -> ("Top"=w70:i32)  [unwired: 2 in, 2 out]
        n130 = property on="Y障礙" class="Bool (strict)"() -> ("Top"=w76:i32)  [unwired: 2 in, 2 out]
        n131 = property on="Y障礙" class="Bool (strict)"() -> ("Left"=w83:i32)  [unwired: 2 in, 2 out]
        n132 = property on="Y障礙" class="Bool (strict)"() -> ("Left"=w81:i32)  [unwired: 2 in, 2 out]
        n133 = Greater?(x=w93, y=250) -> (0:w50:bool)
        n134 = local read "Y"() -> (w84:dbl)
        n135 = local read "X"() -> (w85:dbl)
        n136 = Greater?(x=w44, y=500) -> (0:w42:bool)
        n137 = Add(x=w83, y=17) -> (x+y=w78:i32)
        n138 = Subtract(x=w81, y=17) -> (x-y=w79:i32)
        n139 = Subtract(x=w76, y=15) -> (x-y=w75:i32)
        n140 = Add(x=w70, y=20) -> (x+y=w71:i32)
        n141 = In Range and Coerce(upper limit=w78, x=w85, lower limit=w79) -> (In Range?=w74:bool)  [unwired: 1 out]
        n142 = In Range and Coerce(upper limit=w71, x=w84, lower limit=w75) -> (In Range?=w73:bool)  [unwired: 1 out]
        n143 = And(x=w74, y=w73) -> (x .and. y?=w49:bool)
        n144 = Compound Arithmetic op=OR(w42, w50, w48, w49) -> (w47:bool)
      }
      n145 = call-poly <vilib>:"Close Input Device.vi"("error in (no error)"=w36, "device ID"=w38) -> ()  [unwired: 8 in, 1 out]
    }
    frame #2 {
      w218 = 0.0 ("x*y")
      n146 = Random Number (0-1)() -> (number: 0 to 1=w223:dbl)
      n147 = Random Number (0-1)() -> (number: 0 to 1=w227:dbl)
      n148 = property on="Y障礙" class="Bool (strict)"("Left"=375 ("Position:Left"), "Top"=1 ("Position:Top")) -> ()  [unwired: 2 in, 2 out]
      n149 = local write "Vy"(400 ("Vy")) -> ()
      n150 = local write "Vx"(400 ("Vx")) -> ()
      n151 = Multiply(x=200.0, y=w223) -> (x*y=w221:dbl)
      n152 = Add(x=300.0 ("y"), y=w221) -> (x+y=→"Å]Vy":dbl)
      n153 = local write "y觸及位置"(0 ("y觸及位置")) -> ()
      n154 = local write "x觸及位置"(0 ("x觸及位置")) -> ()
      n155 = Multiply(x=200.0, y=w227) -> (x*y=w225:dbl)
      n156 = Add(x=300.0 ("y"), y=w225) -> (x+y=→"Å]Vx":dbl)
      n157 = property on="X障礙" class="Bool (strict)"("Left"=1 ("Position:Left"), "Top"=340 ("Position:Top")) -> ()  [unwired: 2 in, 2 out]
      "Å]XÄ²" <- w218
      "Å]YÄ²" <- w218
    }
    frame #3 {
      w239 = 0
      w240 = 0
      w250 = 0 ("Top")
      w251 = 0
      n158 = Tick Count (ms)() -> (millisecond timer value=w253:u32)
      n159 = Tick Count (ms)() -> (millisecond timer value=w243:u32)
      n160 = call <vilib>:"Intialize Keyboard.vi"() -> ("error out"=w254:errorcluster, "device ID"=w255:refnum<k1>)  [unwired: 10 in]
      n161 = Tick Count (ms)() -> (millisecond timer value=w242:u32)
      n162 = Tick Count (ms)() -> (millisecond timer value=w256:u32)
      n163 = while {
        shift-right: [w358] -> _
        shift-left: enum16{"speed"}."speed" ("Enum") -> [w360]
        shift-right: [w359] -> _
        shift-left: w256 -> [w361]
        tunnel: w255 -> [w357]
        tunnel: w254 -> [w356]
        shift-right: [w352] -> _
        shift-left: w253 -> [w353]
        shift-right: [w351] -> _
        shift-left: enum16{"speed"}."speed" ("Enum") -> [w350]
        shift-right: [w349] -> _
        shift-left: w251 -> [w348]
        shift-left: w251 -> [w347]
        shift-right: [w346] -> _
        shift-left: w250 -> [w345]
        shift-left: w250 -> [w344]
        tunnel: w249 -> [w342]
        tunnel: w248 -> [w341]
        tunnel: [w324] -> w247
        tunnel: [w323] -> w246
        tunnel: [w293] -> w245
        shift-right: [w286] -> _
        shift-left: w240 -> [w288]
        shift-left: w240 -> [w287]
        shift-right: [w283] -> _
        shift-left: w239 -> [w284]
        shift-left: w239 -> [w285]
        shift-right: [w282] -> _
        shift-left: w243 -> [w291]
        shift-right: [w281] -> _
        shift-left: enum16{"speed"}."speed" ("Enum") -> [w292]
        shift-right: [w280] -> _
        shift-left: w242 -> [w290]
        shift-right: [w279] -> _
        shift-left: enum16{"speed"}."speed" ("Enum") -> [w289]
        stop <- w304 stop-if-true
        # "以下雙方向障礙"
        n164 = local read "遊玩時間"() -> (w302:i32)
        n165 = case shown="\"speed\"" w350 {
          tunnel: w353 -> [w482]
          tunnel: [w480] -> w352
          tunnel: [w479] -> w351
          tunnel: [w463] -> w349
          tunnel: w348 -> [w462]
          tunnel: w348 -> [w461]
          tunnel: w347 -> [w460]
          tunnel: w347 -> [w459]
          frame "speed" {
            n166 = Tick Count (ms)() -> (millisecond timer value=w491:u32)
            n167 = property on="X障礙" class="Bool (strict)"() -> ("Left"=w483:i32)  [unwired: 2 in, 2 out]
            n168 = property on="X障礙" class="Bool (strict)"() -> ("Left"=w477:i32)  [unwired: 2 in, 2 out]
            n169 = Less?(x=w477, y=0) -> (x < y?=w475:bool)
            n170 = Greater?(x=w462, y=500.0) -> (0:w457:bool)
            n171 = Greater?(x=w460, y=500.0) -> (0:w466:bool)
            n172 = Less?(x=w461, y=0.0) -> (x < y?=w469:bool)
            n173 = Less?(x=w459, y=0.0) -> (x < y?=w470:bool)
            n174 = Greater?(x=w483, y=500) -> (0:w474:bool)
            n175 = Subtract(x=w491, y=w482) -> (x-y=w490:u32)
            n176 = Or(x=w474, y=w475) -> (x .or. y?=w473:bool)
            n177 = To Double Precision Float(number=w490) -> (double precision float=w489:dbl)
            n178 = And(x=w457, y=w466) -> (x .and. y?=w471:bool)
            n179 = And(x=w469, y=w470) -> (x .and. y?=w472:bool)
            n180 = Or(x=w471, y=w472) -> (x .or. y?=w458:bool)
            n181 = local read "Vx"() -> (w478:i32)
            n182 = local read "x觸及位置"() -> (w485:i32)
            n183 = Divide(x=w489, y=1000.0) -> (x/y=w487:dbl)
            n184 = case shown="True" w458 {
              frame False {
              }
              frame True {
                w492 = 200 ("x觸及位置")
                n185 = local write "x觸及位置"(w492) -> ()
                n186 = Wait (ms)(milliseconds to wait=u32 100) -> ()  [unwired: 1 out]
                n187 = property on="X障礙" class="Bool (strict)"("Left"=w492) -> ()  [unwired: 2 in, 2 out]
              }
            }
            n188 = Multiply(x=w487, y=w478) -> (x*y=w486:dbl)
            n189 = Add(x=w486, y=w485) -> (x+y=w481:dbl)
            n190 = case shown="True" w473 {
              tunnel: [enum16{"speed"}."speed" ("Enum") enum16{"speed"}."speed" ("Enum")] -> w479
              tunnel: [w494 w501] -> w480
              tunnel: w482 -> [w494 _]
              tunnel: w481 -> [_ w497]
              tunnel: w478 -> [_ w499]
              frame False {
              }
              frame True {
                n191 = local write "x觸及位置"(w497) -> ()
                n192 = Multiply(x=w499, y=-1.0) -> (x*y=w496:dbl)
                n193 = Wait (ms)(milliseconds to wait=u32 25) -> ()  [unwired: 1 out]
                n194 = Tick Count (ms)() -> (millisecond timer value=w501:u32)
                n195 = local write "Vx"(w496) -> ()
              }
            }
            n196 = property on="X障礙" class="Bool (strict)"("Left"=w481) -> ()  [unwired: 2 in, 2 out]
            n197 = Wait (ms)(milliseconds to wait=u32 10) -> ()  [unwired: 1 out]
            n198 = property on="X障礙" class="Bool (strict)"() -> ("Left"=w463:i32)  [unwired: 2 in, 2 out]
          }
        }
        n199 = case shown="\"speed\"" w292 {
          tunnel: w291 -> [w435]
          tunnel: [w433] -> w282
          tunnel: [w432] -> w281
          tunnel: [w416] -> w286
          tunnel: w288 -> [w415]
          tunnel: w288 -> [w414]
          tunnel: w287 -> [w413]
          tunnel: w287 -> [w412]
          frame "speed" {
            n200 = Tick Count (ms)() -> (millisecond timer value=w444:u32)
            n201 = property on="魔王" class="Bool (strict)"() -> ("Left"=w436:i32)  [unwired: 2 in, 2 out]
            n202 = property on="魔王" class="Bool (strict)"() -> ("Left"=w430:i32)  [unwired: 2 in, 2 out]
            n203 = Less?(x=w430, y=0) -> (x < y?=w428:bool)
            n204 = Greater?(x=w415, y=500.0) -> (0:w410:bool)
            n205 = Greater?(x=w413, y=500.0) -> (0:w419:bool)
            n206 = Less?(x=w414, y=0.0) -> (x < y?=w422:bool)
            n207 = Less?(x=w412, y=0.0) -> (x < y?=w423:bool)
            n208 = Greater?(x=w436, y=500) -> (0:w427:bool)
            n209 = Subtract(x=w444, y=w435) -> (x-y=w443:u32)
            n210 = Or(x=w427, y=w428) -> (x .or. y?=w426:bool)
            n211 = To Double Precision Float(number=w443) -> (double precision float=w442:dbl)
            n212 = And(x=w410, y=w419) -> (x .and. y?=w424:bool)
            n213 = And(x=w422, y=w423) -> (x .and. y?=w425:bool)
            n214 = Or(x=w424, y=w425) -> (x .or. y?=w411:bool)
            n215 = local read "Å]Vx"() -> (w431:i32)
            n216 = Divide(x=w442, y=1000.0) -> (x/y=w440:dbl)
            n217 = local read "Å]XÄ²"() -> (w438:i32)
            n218 = case shown="True" w411 {
              frame False {
              }
              frame True {
                w445 = 200 ("x觸及位置")
                n219 = local write "Å]XÄ²"(w445) -> ()
                n220 = Wait (ms)(milliseconds to wait=u32 100) -> ()  [unwired: 1 out]
                n221 = property on="魔王" class="Bool (strict)"("Left"=w445) -> ()  [unwired: 2 in, 2 out]
              }
            }
            n222 = Multiply(x=w440, y=w431) -> (x*y=w439:dbl)
            n223 = Add(x=w439, y=w438) -> (x+y=w434:dbl)
            n224 = case shown="True" w426 {
              tunnel: [enum16{"speed"}."speed" ("Enum") enum16{"speed"}."speed" ("Enum")] -> w432
              tunnel: [w447 w454] -> w433
              tunnel: w435 -> [w447 _]
              tunnel: w434 -> [_ w450]
              tunnel: w431 -> [_ w452]
              frame False {
              }
              frame True {
                n225 = Multiply(x=w452, y=-1.0) -> (x*y=w449:dbl)
                n226 = local write "Å]XÄ²"(w450) -> ()
                n227 = Wait (ms)(milliseconds to wait=u32 25) -> ()  [unwired: 1 out]
                n228 = local write "Å]Vx"(w449) -> ()
                n229 = Tick Count (ms)() -> (millisecond timer value=w454:u32)
              }
            }
            n230 = property on="魔王" class="Bool (strict)"("Left"=w434) -> ()  [unwired: 2 in, 2 out]
            n231 = Wait (ms)(milliseconds to wait=u32 10) -> ()  [unwired: 1 out]
            n232 = property on="魔王" class="Bool (strict)"() -> ("Left"=w416:i32)  [unwired: 2 in, 2 out]
          }
        }
        n233 = case shown="\"speed\"" w289 {
          tunnel: w290 -> [w388]
          tunnel: [w386] -> w280
          tunnel: [w385] -> w279
          tunnel: [w369] -> w283
          tunnel: w285 -> [w368]
          tunnel: w285 -> [w367]
          tunnel: w284 -> [w366]
          tunnel: w284 -> [w365]
          frame "speed" {
            n234 = Tick Count (ms)() -> (millisecond timer value=w397:u32)
            n235 = property on="魔王" class="Bool (strict)"() -> ("Top"=w389:i32)  [unwired: 2 in, 2 out]
            n236 = property on="魔王" class="Bool (strict)"() -> ("Top"=w383:i32)  [unwired: 2 in, 2 out]
            n237 = Less?(x=w383, y=0) -> (x < y?=w381:bool)
            n238 = Greater?(x=w368, y=400.0) -> (0:w363:bool)
            n239 = Greater?(x=w366, y=400.0) -> (0:w372:bool)
            n240 = Less?(x=w367, y=0.0) -> (x < y?=w375:bool)
            n241 = Less?(x=w365, y=0.0) -> (x < y?=w376:bool)
            n242 = Greater?(x=w389, y=400) -> (0:w380:bool)
            n243 = Subtract(x=w397, y=w388) -> (x-y=w396:u32)
            n244 = Or(x=w380, y=w381) -> (x .or. y?=w379:bool)
            n245 = To Double Precision Float(number=w396) -> (double precision float=w395:dbl)
            n246 = And(x=w363, y=w372) -> (x .and. y?=w377:bool)
            n247 = And(x=w375, y=w376) -> (x .and. y?=w378:bool)
            n248 = Or(x=w377, y=w378) -> (x .or. y?=w364:bool)
            n249 = local read "Å]Vy"() -> (w384:i64)
            n250 = Divide(x=w395, y=1000.0) -> (x/y=w393:dbl)
            n251 = local read "Å]YÄ²"() -> (w391:i32)
            n252 = case shown="True" w364 {
              frame False {
              }
              frame True {
                w398 = 200 ("x觸及位置")
                n253 = local write "Å]YÄ²"(w398) -> ()
                n254 = Wait (ms)(milliseconds to wait=u32 100) -> ()  [unwired: 1 out]
                n255 = property on="魔王" class="Bool (strict)"("Top"=w398) -> ()  [unwired: 2 in, 2 out]
              }
            }
            n256 = Multiply(x=w393, y=w384) -> (x*y=w392:dbl)
            n257 = Add(x=w392, y=w391) -> (x+y=w387:dbl)
            n258 = case shown="True" w379 {
              tunnel: [enum16{"speed"}."speed" ("Enum") enum16{"speed"}."speed" ("Enum")] -> w385
              tunnel: [w400 w407] -> w386
              tunnel: w388 -> [w400 _]
              tunnel: w387 -> [_ w403]
              tunnel: w384 -> [_ w405]
              frame False {
              }
              frame True {
                n259 = Multiply(x=w405, y=-1.0) -> (x*y=w402:dbl)
                n260 = local write "Å]YÄ²"(w403) -> ()
                n261 = Wait (ms)(milliseconds to wait=u32 25) -> ()  [unwired: 1 out]
                n262 = local write "Å]Vy"(w402) -> ()
                n263 = Tick Count (ms)() -> (millisecond timer value=w407:u32)
              }
            }
            n264 = property on="魔王" class="Bool (strict)"("Top"=w387) -> ()  [unwired: 2 in, 2 out]
            n265 = Wait (ms)(milliseconds to wait=u32 10) -> ()  [unwired: 1 out]
            n266 = property on="魔王" class="Bool (strict)"() -> ("Top"=w369:i32)  [unwired: 2 in, 2 out]
          }
        }
        n267 = case shown="\"speed\"" w360 {
          tunnel: w361 -> [w545]
          tunnel: [w543] -> w359
          tunnel: [w542] -> w358
          tunnel: [w526] -> w346
          tunnel: w345 -> [w525]
          tunnel: w345 -> [w524]
          tunnel: w344 -> [w523]
          tunnel: w344 -> [w522]
          frame "speed" {
            n268 = Tick Count (ms)() -> (millisecond timer value=w554:u32)
            n269 = Greater?(x=w525, y=400.0) -> (0:w520:bool)
            n270 = Greater?(x=w523, y=400.0) -> (0:w529:bool)
            n271 = Less?(x=w524, y=0.0) -> (x < y?=w532:bool)
            n272 = Less?(x=w522, y=0.0) -> (x < y?=w533:bool)
            n273 = property on="Y障礙" class="Bool (strict)"() -> ("Top"=w546:i32)  [unwired: 2 in, 2 out]
            n274 = property on="Y障礙" class="Bool (strict)"() -> ("Top"=w540:i32)  [unwired: 2 in, 2 out]
            n275 = Less?(x=w540, y=0) -> (x < y?=w538:bool)
            n276 = Greater?(x=w546, y=400) -> (0:w537:bool)
            n277 = Subtract(x=w554, y=w545) -> (x-y=w553:u32)
            n278 = Or(x=w537, y=w538) -> (x .or. y?=w536:bool)
            n279 = And(x=w520, y=w529) -> (x .and. y?=w534:bool)
            n280 = And(x=w532, y=w533) -> (x .and. y?=w535:bool)
            n281 = To Double Precision Float(number=w553) -> (double precision float=w552:dbl)
            n282 = Or(x=w534, y=w535) -> (x .or. y?=w521:bool)
            n283 = local read "Vy"() -> (w541:i32)
            n284 = local read "y觸及位置"() -> (w548:i32)
            n285 = Divide(x=w552, y=1000.0) -> (x/y=w550:dbl)
            n286 = case shown="True" w521 {
              frame False {
              }
              frame True {
                w555 = 200 ("y觸及位置")
                n287 = local write "y觸及位置"(w555) -> ()
                n288 = Wait (ms)(milliseconds to wait=u32 100) -> ()  [unwired: 1 out]
                n289 = property on="Y障礙" class="Bool (strict)"("Top"=w555) -> ()  [unwired: 2 in, 2 out]
              }
            }
            n290 = Multiply(x=w550, y=w541) -> (x*y=w549:dbl)
            n291 = Add(x=w549, y=w548) -> (x+y=w544:dbl)
            n292 = case shown="True" w536 {
              tunnel: [enum16{"speed"}."speed" ("Enum") enum16{"speed"}."speed" ("Enum")] -> w542
              tunnel: [w557 w564] -> w543
              tunnel: w545 -> [w557 _]
              tunnel: w544 -> [_ w560]
              tunnel: w541 -> [_ w562]
              frame False {
              }
              frame True {
                n293 = local write "y觸及位置"(w560) -> ()
                n294 = Multiply(x=w562, y=-1.0) -> (x*y=w559:dbl)
                n295 = Wait (ms)(milliseconds to wait=u32 25) -> ()  [unwired: 1 out]
                n296 = Tick Count (ms)() -> (millisecond timer value=w564:u32)
                n297 = local write "Vy"(w559) -> ()
              }
            }
            n298 = property on="Y障礙" class="Bool (strict)"("Top"=w544) -> ()  [unwired: 2 in, 2 out]
            n299 = property on="Y障礙" class="Bool (strict)"() -> ("Top"=w526:i32)  [unwired: 2 in, 2 out]
            n300 = Wait (ms)(milliseconds to wait=u32 10) -> ()  [unwired: 1 out]
          }
        }
        n301 = call-poly <vilib>:"Acquire Input Data.vi"("device ID"=w357, "error in (no error)"=w356) -> ("device ID"=w324:refnum<k1>, "keys pressed"=w355:T1, "error out"=w323:errorcluster)  [unwired: 15 in]
        n302 = Increment(x=w302) -> (x+1=w303:i32)
        n303 = local write "遊玩時間"(w303) -> ()
        n304 = Array To Cluster(array=w355) -> (cluster=w343:T2)
        n305 = Unbundle(w343) -> ("keys pressed[0]"=w354:T3)  [unwired: 8 out]
        n306 = case shown="\"A\"" w354 {
          frame Default {
          }
          frame "A" {
            n307 = local read "X"() -> (w517:dbl)
            n308 = Wait (ms)(milliseconds to wait=u32 10) -> ()  [unwired: 1 out]
            n309 = Add(x=-2.0, y=w517) -> (x+y=w515:dbl)
            n310 = local write "X"(w515) -> ()
            n311 = property on="小精靈" class="Bool (strict)"("Left"=w515) -> ()  [unwired: 2 in, 2 out]
          }
        }
        n312 = case shown="\"D\"" w354 {
          frame Default {
          }
          frame "D" {
            n313 = local read "X"() -> (w513:dbl)
            n314 = Wait (ms)(milliseconds to wait=u32 10) -> ()  [unwired: 1 out]
            n315 = Add(x=2.0, y=w513) -> (x+y=w511:dbl)
            n316 = local write "X"(w511) -> ()
            n317 = property on="小精靈" class="Bool (strict)"("Left"=w511) -> ()  [unwired: 2 in, 2 out]
          }
        }
        n318 = property on="Y障礙" class="Bool (strict)"() -> ("Top"=w325:i32)  [unwired: 2 in, 2 out]
        n319 = property on="Y障礙" class="Bool (strict)"() -> ("Top"=w331:i32)  [unwired: 2 in, 2 out]
        n320 = property on="Y障礙" class="Bool (strict)"() -> ("Left"=w338:i32)  [unwired: 2 in, 2 out]
        n321 = property on="Y障礙" class="Bool (strict)"() -> ("Left"=w336:i32)  [unwired: 2 in, 2 out]
        n322 = case shown="\"W\"" w354 {
          frame Default {
          }
          frame "W" {
            n323 = local read "Y"() -> (w509:dbl)
            n324 = Wait (ms)(milliseconds to wait=u32 10) -> ()  [unwired: 1 out]
            n325 = Add(x=-2.0, y=w509) -> (x+y=w507:dbl)
            n326 = local write "Y"(w507) -> ()
            n327 = property on="小精靈" class="Bool (strict)"("Top"=w507) -> ()  [unwired: 2 in, 2 out]
          }
        }
        n328 = case shown="\"S\"" w354 {
          frame Default {
          }
          frame "S" {
            n329 = local read "Y"() -> (w505:dbl)
            n330 = Wait (ms)(milliseconds to wait=u32 10) -> ()  [unwired: 1 out]
            n331 = Add(x=2.0, y=w505) -> (x+y=w503:dbl)
            n332 = local write "Y"(w503) -> ()
            n333 = property on="小精靈" class="Bool (strict)"("Top"=w503) -> ()  [unwired: 2 in, 2 out]
          }
        }
        n334 = local read "Y"() -> (w339:dbl)
        n335 = local read "X"() -> (w340:dbl)
        n336 = Add(x=w338, y=17) -> (x+y=w333:i32)
        n337 = Subtract(x=w336, y=17) -> (x-y=w334:i32)
        n338 = Subtract(x=w331, y=15) -> (x-y=w330:i32)
        n339 = Add(x=w325, y=20) -> (x+y=w326:i32)
        n340 = In Range and Coerce(upper limit=w333, x=w340, lower limit=w334) -> (In Range?=w329:bool)  [unwired: 1 out]
        n341 = In Range and Coerce(upper limit=w326, x=w339, lower limit=w330) -> (In Range?=w328:bool)  [unwired: 1 out]
        n342 = And(x=w329, y=w328) -> (x .and. y?=w322:bool)
        n343 = property on="X障礙" class="Bool (strict)"() -> ("Top"=w321:i32)  [unwired: 2 in, 2 out]
        n344 = property on="X障礙" class="Bool (strict)"() -> ("Top"=w315:i32)  [unwired: 2 in, 2 out]
        n345 = property on="X障礙" class="Bool (strict)"() -> ("Left"=w308:i32)  [unwired: 2 in, 2 out]
        n346 = property on="X障礙" class="Bool (strict)"() -> ("Left"=w310:i32)  [unwired: 2 in, 2 out]
        n347 = local read "Y"() -> (w307:dbl)
        n348 = property on="魔王" class="Bool (strict)"() -> ("Top"=w263:i32)  [unwired: 2 in, 2 out]
        n349 = property on="魔王" class="Bool (strict)"() -> ("Top"=w269:i32)  [unwired: 2 in, 2 out]
        n350 = property on="魔王" class="Bool (strict)"() -> ("Left"=w276:i32)  [unwired: 2 in, 2 out]
        n351 = property on="魔王" class="Bool (strict)"() -> ("Left"=w274:i32)  [unwired: 2 in, 2 out]
        n352 = local read "X"() -> (w306:dbl)
        n353 = local read "Y"() -> (w277:dbl)
        n354 = local read "X"() -> (w278:dbl)
        n355 = local read "X"() -> (w301:dbl)
        n356 = local read "Y"() -> (w300:dbl)
        n357 = Add(x=w308, y=17) -> (x+y=w313:i32)
        n358 = Subtract(x=w310, y=17) -> (x-y=w312:i32)
        n359 = Subtract(x=w315, y=15) -> (x-y=w316:i32)
        n360 = Add(x=w321, y=20) -> (x+y=w320:i32)
        n361 = Add(x=w276, y=17) -> (x+y=w271:i32)
        n362 = Subtract(x=w274, y=17) -> (x-y=w272:i32)
        n363 = Subtract(x=w269, y=15) -> (x-y=w268:i32)
        n364 = Add(x=w263, y=20) -> (x+y=w264:i32)
        n365 = In Range and Coerce(upper limit=w313, x=w306, lower limit=w312) -> (In Range?=w317:bool)  [unwired: 1 out]
        n366 = In Range and Coerce(upper limit=w320, x=w307, lower limit=w316) -> (In Range?=w318:bool)  [unwired: 1 out]
        n367 = In Range and Coerce(upper limit=516.0, x=w301, lower limit=463.0) -> (In Range?=w299:bool)  [unwired: 1 out]
        n368 = In Range and Coerce(upper limit=399.0, x=w300, lower limit=358.0) -> (In Range?=w298:bool)  [unwired: 1 out]
        n369 = In Range and Coerce(upper limit=w271, x=w278, lower limit=w272) -> (In Range?=w267:bool)  [unwired: 1 out]
        n370 = In Range and Coerce(upper limit=w264, x=w277, lower limit=w268) -> (In Range?=w266:bool)  [unwired: 1 out]
        n371 = And(x=w317, y=w318) -> (x .and. y?=w305:bool)
        n372 = And(x=w299, y=w298) -> (x .and. y?=w293:bool)
        n373 = And(x=w267, y=w266) -> (x .and. y?=w262:bool)
        n374 = Compound Arithmetic op=OR(w262, w342, w341, w322, w305, w293) -> (w304:bool)
      }
      "高難度挑戰" <- w245
      n375 = call-poly <vilib>:"Close Input Device.vi"("error in (no error)"=w246, "device ID"=w247) -> ()  [unwired: 8 in, 1 out]
      n376 = case shown="True" w245 {
        frame False {
          n377 = One Button Dialog(message="你也太爛了吧", button name ("OK")="對") -> ()  [unwired: 1 out]
        }
        frame True {
          n378 = One Button Dialog(message="復健成功", button name ("OK")="再來啊!") -> ()  [unwired: 1 out]
        }
      }
    }
  }
  "終點" <- TRUE ("Boolean 3")
